vi "instrumentProperties_gainLevels_available.vi"(0 "reference":refnum<class "OSA200.lvclass">, 5 "error in (no error)":errorcluster) -> (10 "status":string, 14 "duplicate reference":refnum<class "OSA200.lvclass">, 16 "gainLevels out":dbl[](array[numeric]), 19 "error out":errorcluster)   [LabVIEW 2010, in "OSA200.lvclass"]
doc: "Resolution depends on resolution mode."
uses:
  OSA200.lvclass
  OSA.lvclass
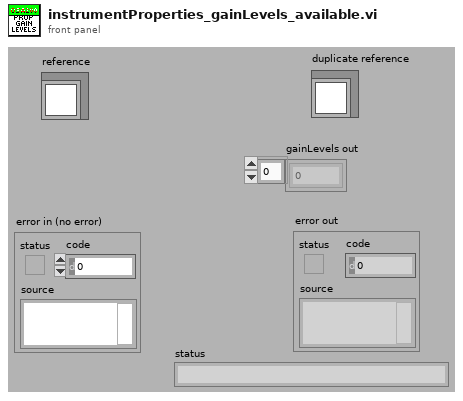
[diagram p1: front panel]
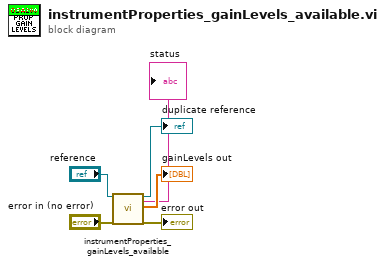
[diagram p0: block diagram]
diagram:
  n1 = call-parent "instrumentProperties_gainLevels_available.vi"("reference"="reference", "error in (no error)"="error in (no error)") -> ("status"=→"status":string, "duplicate reference"=→"duplicate reference":refnum<class "OSA200.lvclass">, "gainLevels out"=→"gainLevels out":dbl[], "error out"=→"error out":errorcluster)  [unwired: 14 in]
